vi "GOMDBTS2048 get CRI.vi"(0 "handle":i32, 7 "error in (no error)":errorcluster) -> (10 "R15":dbl, 11 "function return":i32, 12 "R13":dbl, 13 "R14":dbl, 14 "R11":dbl, 15 "R12":dbl, 16 "R9":dbl, 17 "R10":dbl, 18 "R7":dbl, 19 "R8":dbl, 20 "Ra":dbl, 21 "R1":dbl, 22 "R2":dbl, 23 "R3":dbl, 24 "R4":dbl, 25 "R5":dbl, 26 "R6":dbl, 27 "error out":errorcluster)   [LabVIEW 2015, in "GOMDBTS2048.lvlib"]
doc: "GOBTS2048DLL int __stdcall GOMDBTS2048_getCRI(int handle, double* Ra, double* R1, double* R2, double* R3, double* R4, double* R5, double* R6,\n double* R7, double* R8, double* R9, double* R10, double* R11, double* R12, double* R13, double* R14, double* R15);"
uses:
  GOMDBTS2048.lvlib
  runtime/GOMDBTS2048.dll
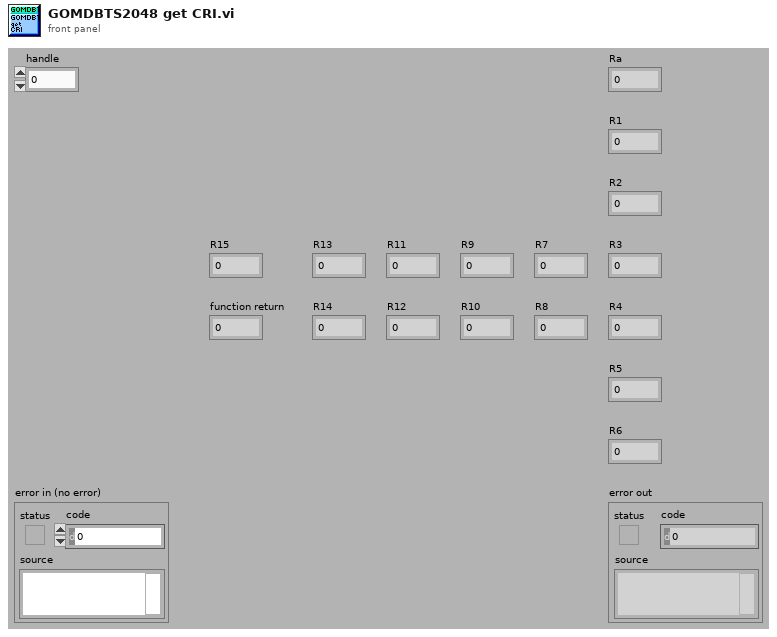
[diagram p1: front panel]
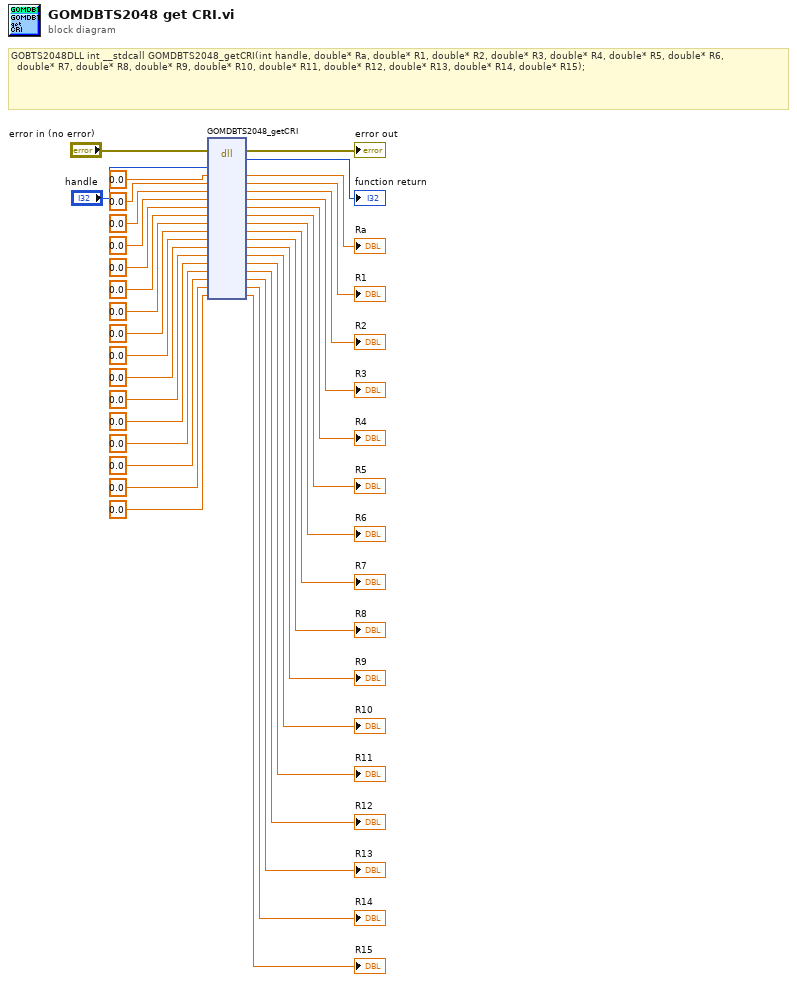
[diagram p0: block diagram]
diagram:
  # "GOBTS2048DLL int __stdcall GOMDBTS2048_getCRI(int handle, double* Ra, double* R1, double* R2, double* R3, double* R4, double* R5, double* R6,\n\t\tdouble* R7, double* R8, double* R9, double* R10, double* R11, double* R12, double* R13, double* R14, double* R15);"
  n1 = dll-call lib="C:/Users/rkoch/Documents/GO_Library/runtime/GOMDBTS2048.*" fn="GOMDBTS2048_getCRI"(error in="error in (no error)", "handle"="handle", "Ra"=0.0, "R1"=0.0, "R2"=0.0, "R3"=0.0, "R4"=0.0, "R5"=0.0, "R6"=0.0, "R7"=0.0, "R8"=0.0, "R9"=0.0, "R10"=0.0, "R11"=0.0, "R12"=0.0, "R13"=0.0, "R14"=0.0, "R15"=0.0) -> (error out=→"error out":errorcluster, →"function return":i32, "Ra"=→"Ra":dbl, "R1"=→"R1":dbl, "R2"=→"R2":dbl, "R3"=→"R3":dbl, "R4"=→"R4":dbl, "R5"=→"R5":dbl, "R6"=→"R6":dbl, "R7"=→"R7":dbl, "R8"=→"R8":dbl, "R9"=→"R9":dbl, "R10"=→"R10":dbl, "R11"=→"R11":dbl, "R12"=→"R12":dbl, "R13"=→"R13":dbl, "R14"=→"R14":dbl, "R15"=→"R15":dbl)  [unwired: 3 in, 1 out]
